vi "BRig_dataExp_Cue2Switch_Prob_PostR.vi"() -> (2 "output_Cue2Switch_Prob_PostR":i32)   [LabVIEW 2014]
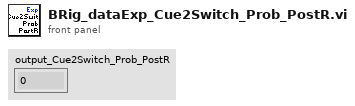
[diagram p1: front panel]
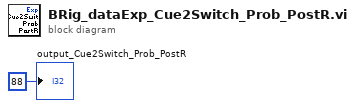
[diagram p0: block diagram]
diagram:
  "output_Cue2Switch_Prob_PostR" <- 88 ("output_iBlock")
